vi "Draw.vi"(8 "error in (no error)":errorcluster, 11 "Menu in":refnum<class "Menu.lvclass">) -> (0 "error out":errorcluster, 3 "Menu out":refnum<class "Menu.lvclass">)   [LabVIEW 2019, in "RT_Game.lvlib" / "Menu.lvclass"]
uses:
  Menu.lvclass
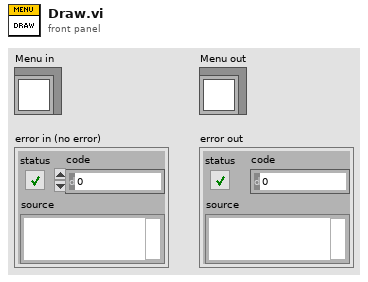
[diagram p1: front panel]
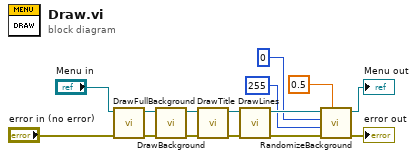
[diagram p0: block diagram]
diagram:
  n1 = call "DrawFullBackground.vi"("error in (no error)"="error in (no error)", "Menu in"="Menu in") -> ("error out"=w9:errorcluster, "Menu out"=w7:refnum<class "Menu.lvclass">)  [unwired: 8 in]
  n2 = call "DrawBackground.vi"("error in (no error)"=w9, "Menu in"=w7) -> ("error out"=w11:errorcluster, "Menu out"=w13:refnum<class "Menu.lvclass">)  [unwired: 8 in]
  n3 = call "DrawTitle.vi"("error in (no error)"=w11, "Menu in"=w13) -> ("error out"=w12:errorcluster, "Menu out"=w14:refnum<class "Menu.lvclass">)  [unwired: 8 in]
  n4 = call "DrawLines.vi"("error in (no error)"=w12, "Menu in"=w14) -> ("error out"=w8:errorcluster, "Menu out"=w5:refnum<class "Menu.lvclass">)  [unwired: 8 in]
  n5 = call "RandomizeBackground.vi"("Possibility"=0.5, "error in (no error)"=w8, "ReplaceTilecode"=u8 255, "ToReplaceTilecode"=u8 0, "Menu in"=w5) -> ("error out"=→"error out":errorcluster, "Menu out"=→"Menu out":refnum<class "Menu.lvclass">)  [unwired: 5 in]
